vi "0816147.vi"() -> ()   [LabVIEW 2021]
panel:
  in  "Numeric":dbl
  out "point":bool
  out "0.1":T1
  out "1":T1
  out "10":T1
  out "100":T1
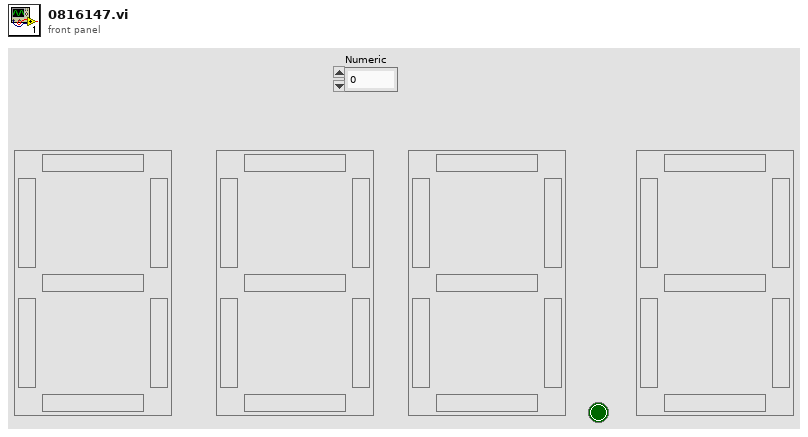
[diagram p1: front panel]
types:
  T1 = cluster{"Boolean 1":bool, "Boolean 2":bool, "Boolean 3":bool, "Boolean 4":bool, "Boolean 5":bool, "Boolean 6":bool, "Boolean 7":bool}
  T2 = cluster{"[0]":bool, "[1]":bool, "[2]":bool, "[3]":bool, "[4]":bool, "[5]":bool, "[6]":bool}
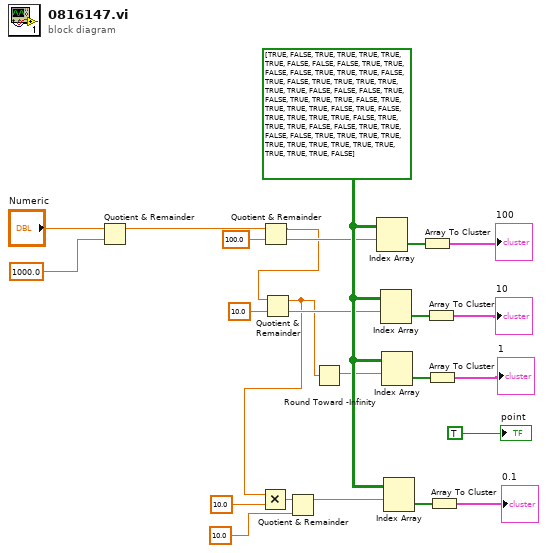
[diagram p0: block diagram]
diagram:
  w19 = bool[][] [[TRUE, FALSE, TRUE, TRUE, TRUE, TRUE, TRUE], [FALSE, FALSE, FALSE, TRUE, TRUE, FALSE, FALSE], [TRUE, TRUE, TRUE, FALSE, TRUE, FALSE, TRUE], [TRUE, TRUE, TRUE, TRUE, TRUE, FALSE, FALSE], [FALSE, TRUE, FALSE, TRUE, TRUE, TRUE, FALSE], [TRUE, TRUE, TRUE, TRUE, FALSE, TRUE, FALSE], [TRUE, TRUE, TRUE, TRUE, FALSE, TRUE, TRUE], [TRUE, FALSE, FALSE, TRUE, TRUE, FALSE, FALSE], [TRUE, TRUE, TRUE, TRUE, TRUE, TRUE, TRUE], [TRUE, TRUE, TRUE, TRUE, TRUE, TRUE, FALSE]]
  n1 = Quotient & Remainder(x="Numeric", y=1000.0) -> (x-y*floor(x/y)=w2:dbl)  [unwired: 1 out]
  n2 = Quotient & Remainder(x=w2, y=100.0) -> (x-y*floor(x/y)=w11:dbl, floor(x/y)=w14:dbl)
  n3 = Quotient & Remainder(x=w11, y=10.0) -> (x-y*floor(x/y)=w5:dbl, floor(x/y)=w13:dbl)
  n4 = Multiply(x=w5, y=10.0) -> (x*y=w7:dbl)
  n5 = Quotient & Remainder(x=w7, y=10.0) -> (x-y*floor(x/y)=w9:dbl)  [unwired: 1 out]
  n6 = Round Toward -Infinity(1:w5) -> (0:w6:dbl)
  n7 = Index Array(array=w19, index (row)=w14) -> (element=w24:bool[])  [unwired: 1 in]
  n8 = Index Array(array=w19, index (row)=w13) -> (element=w22:bool[])  [unwired: 1 in]
  n9 = Index Array(array=w19, index (row)=w6) -> (element=w21:bool[])  [unwired: 1 in]
  n10 = Index Array(array=w19, index (row)=w9) -> (element=w20:bool[])  [unwired: 1 in]
  n11 = Array To Cluster(array=w24) -> (cluster=→"100":T2)
  n12 = Array To Cluster(array=w22) -> (cluster=→"10":T2)
  n13 = Array To Cluster(array=w21) -> (cluster=→"1":T2)
  n14 = Array To Cluster(array=w20) -> (cluster=→"0.1":T2)
  "point" <- TRUE ("point")
